vi "Check Embedded.vi"(7 "SVG Path":path, 9 "error in (no error)":errorcluster, 11 "URI":string) -> (1 "error out":errorcluster, 2 "Embedded":bool, 3 "Path Out":string)   [LabVIEW 2019, in "SVGImage.lvclass"]
uses:
  SVGImage.lvclass
  <vilib>/LabVIEW Open Source Project/OpenURI/utilities/Extract URI Components.vi
  <vilib>/LabVIEW Open Source Project/OpenURI/openURI.lvlib
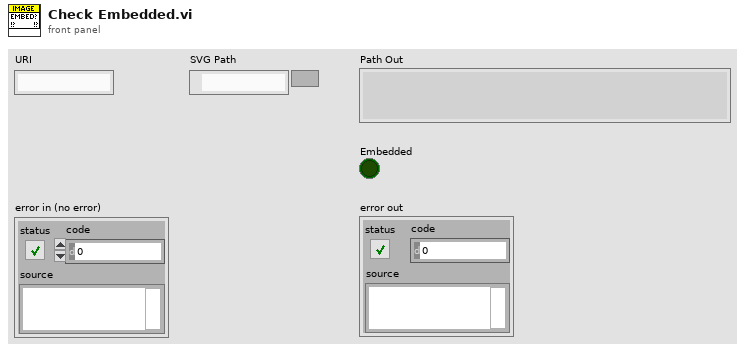
[diagram p1: front panel]
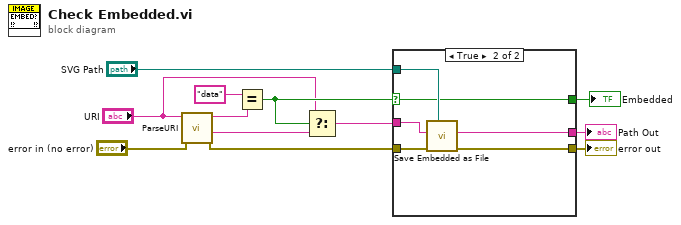
[diagram p0: block diagram]
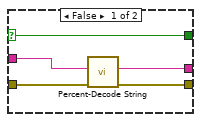
[diagram p2: hidden frame]
diagram:
  n1 = call <vilib>:"ParseURI.vi"("error in"="error in (no error)", "URI"="URI") -> ("error out"=w8:errorcluster, "path"=w1:string, "scheme"=w12:string)  [unwired: 4 in, 3 out]
  n2 = Equal?(x="data", y=w12) -> (x = y?=w4:bool)
  n3 = Select(t="URI", s=w4, f=w1) -> (s? t:f=w2:string)
  n4 = case shown="True" w4 {
    selector: w4 -> [w13 w18]
    tunnel: w2 -> [w16 w17]
    tunnel: [w15 w19] -> w10
    tunnel: "SVG Path" -> [_ w20]
    tunnel: w8 -> [w14 w22]
    tunnel: [w14 w21] -> w7
    tunnel: [w13 w18] -> w5
    frame False {
      n5 = call <vilib>:"Percent-Decode String.vi"("Pct-Encoded String"=w16) -> ("String"=w15:string)  [unwired: 10 in]
    }
    frame True {
      n6 = call "Save Embedded as File.vi"("Inkscape Path"=w20, "error in (no error)"=w22, "Base64 Encoded String"=w17) -> ("error out"=w21:errorcluster, "Path Out"=w19:string)  [unwired: 7 in]
    }
  }
  "Embedded" <- w5
  "Path Out" <- w10
  "error out" <- w7
